vi "Read Handler Input Data.vi"(8 "error in (no error)":errorcluster, 10 "Port (0: C)":u16(ring) items=["C", "D", "E", "F", "G", "H", "A", "B", "C"], 11 "VISA resource name":refnum<visa-resource-name>) -> (0 "error out":errorcluster, 2 "Data":i32, 3 "VISA resource name out":refnum<visa-resource-name>)   [LabVIEW 2020, in "Agilent ENA Series.lvlib"]
doc: "Reads out data inputted to ports C, D or E (C0 to\nC3, D0 to D3 or C0 to D3).\n\nNotes:\n(1) Ports C or D must be set to input mode for read out from the port C or D.\n(2) Ports C and D must be set to input mode for read out from the port E."
uses:
  <instrlib>/Agilent ENA Series/Agilent ENA Series.lvlib
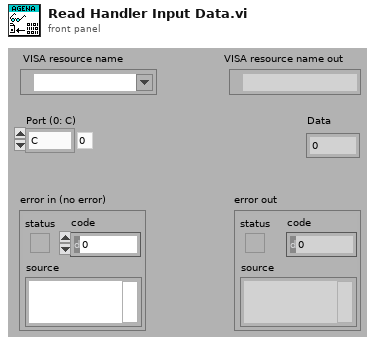
[diagram p1: front panel]
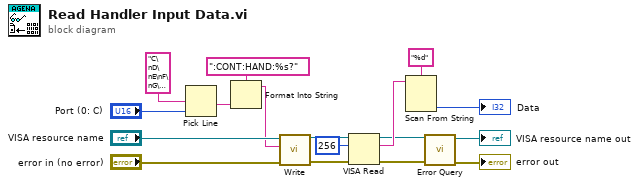
[diagram p0: block diagram]
diagram:
  n1 = Pick Line(multi-line string="C\nD\nE\nF\nG\nH\nA\nB\nC", line index="Port (0: C)") -> (output string=w11:string)  [unwired: 1 in]
  n2 = Format Into String(format string=":CONT:HAND:%s?", w11) -> (resulting string=w14:string)  [unwired: 2 in, 1 out]
  n3 = call <instrlib>:"Write.vi"("error in (no error)"="error in (no error)", "String ()"=w14, "VISA resource name"="VISA resource name") -> ("error out"=w9:errorcluster, "VISA resource name out"=w10:refnum<visa-resource-name>)  [unwired: 6 in, 1 out]
  n4 = VISA Read(VISA resource name=w10, byte count=u32 256, error in (no error)=w9) -> (VISA resource name out=w4:refnum<visa-resource-name>, read buffer=w6:string, error out=w3:errorcluster)  [unwired: 1 out]
  n5 = Scan From String(format string="%d", input string=w6) -> (output 1=→"Data":i32)  [unwired: 3 in, 3 out]
  n6 = call <instrlib>:"Error Query.vi"("error in (no error)"=w3, "VISA resource name"=w4) -> ("error out"=→"error out":errorcluster, "VISA resource name out"=→"VISA resource name out":refnum<visa-resource-name>)  [unwired: 6 in, 2 out]
